vi "OpenCreateVI.vi"(8 "error in":errorcluster, 11 "State":T1) -> (0 "error out":errorcluster, 3 "State out":T1)   [LabVIEW 2013, in "control module data interface generator.lvlib"]
uses:
  control module data interface generator.lvlib
  Controls/StateCluster.ctl
  Controls/initialized references.ctl
  Controls/interface VI type.ctl
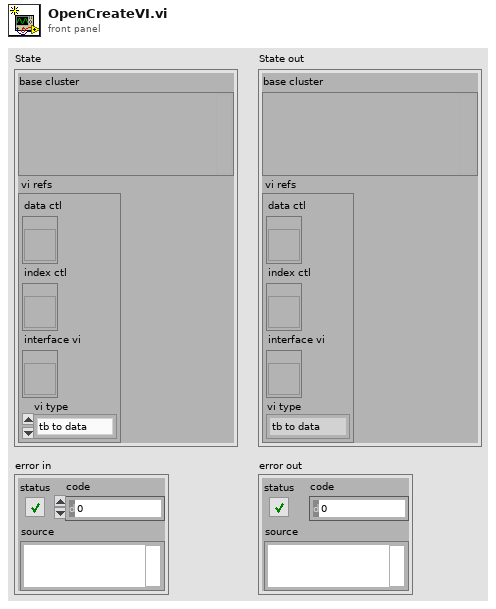
[diagram p1: front panel]
types:
  T1 = typedef "control module data interface generator.lvlib/StateCluster.ctl" = cluster{"base cluster":variant, "vi refs":T2}
  T2 = typedef "control module data interface generator.lvlib/initialized references.ctl" = cluster{"data ctl":refnum<vi>, "index ctl":refnum<vi>, "interface vi":refnum<vi>, "vi type":T3}
  T3 = typedef "control module data interface generator.lvlib/interface VI type.ctl" = enum16{"tb to data", "data to tb"}
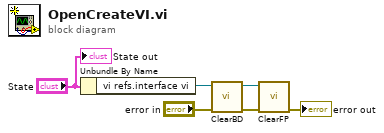
[diagram p0: block diagram]
diagram:
  n1 = Unbundle By Name("State") -> ("vi refs.interface vi"=w2:refnum<vi>)
  n2 = call "ClearBD.vi"("error in"="error in", "reference"=w2) -> ("error out"=w6:errorcluster, "reference out"=w5:refnum<vi>)  [unwired: 8 in]
  n3 = call "ClearFP.vi"("error in"=w6, "reference"=w5) -> ("error out"=→"error out":errorcluster)  [unwired: 8 in, 1 out]
  "State out" <- "State"
